vi "Initiate Syringe Home.vi"(8 "error in (no error)":errorcluster) -> (0 "error out":errorcluster)   [LabVIEW 2015, in "cRIO-Carbondioxide.lvlib" / "cRIO-CO2.lvlib" / "cRIO-CO2.lvclass"]
uses:
  cRIO-CO2.lvclass
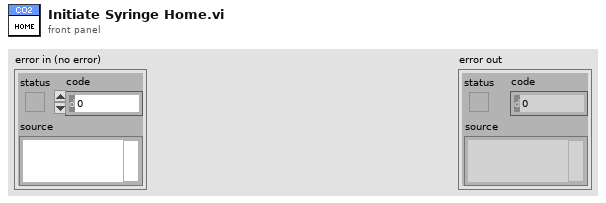
[diagram p1: front panel]
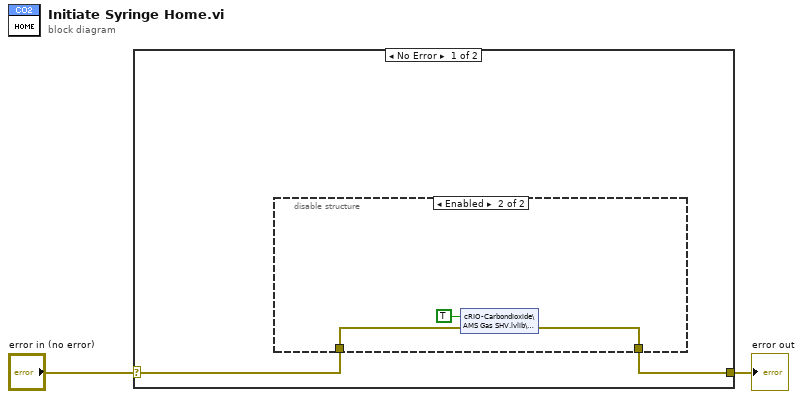
[diagram p0: block diagram]
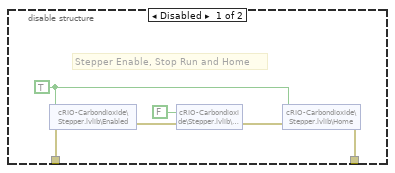
[diagram p2: hidden frame]
diagram:
  n1 = case shown="No Error" "error in (no error)" {
    selector: "error in (no error)" -> [w4 w14]
    tunnel: [w3 w14] -> w1
    frame No Error {
      n2 = disable-structure shown="Enabled" {
        disable-tunnel: w4 -> [w9 w13]
        disable-tunnel: [w8 w12] -> w3
        frame Disabled {
          w10 = TRUE ("Enabled")
          # "Stepper Enable, Stop Run and Home"
          n3 = shared-variable "cRIO-Carbondioxide\\Stepper.lvlib\\Enabled"(w10, error in=w9) -> (error out=w7:errorcluster)
          n4 = shared-variable "cRIO-Carbondioxide\\Stepper.lvlib\\Run"(FALSE ("Run"), error in=w7) -> (error out=w6:errorcluster)
          n5 = shared-variable "cRIO-Carbondioxide\\Stepper.lvlib\\Home"(w10, error in=w6) -> (error out=w8:errorcluster)
        }
        frame Enabled {
          n6 = shared-variable "cRIO-Carbondioxide\\AMS Gas SHV.lvlib\\Cylinder.lvlib\\Home"(TRUE ("Home"), error in=w13) -> (error out=w12:errorcluster)
        }
      }
    }
    frame Error {
    }
  }
  "error out" <- w1
